vi "FT_Get_Device_Serial_Number_By_Index2011.vi"(0 "Device Index":u32) -> (1 "FT_Status":u32(ring) items=["FT_OK", "FT_INVALID_HANDLE", "FT_DEVICE_NOT_FOUND", "FT_DEVICE_NOT_OPENED", "FT_IO_ERROR", "FT_INSUFFICIENT_RESOURCES", "FT_INVALID_PARAMETER", "FT_INVALID_BAUD_RATE", "FT_DEVICE_NOT_OPENED_FOR_ERASE", "FT_DEVICE_NOT_OPENED_FOR_WRITE", "FT_FAILED_TO_WRITE_DEVICE", "FT_EEPROM_READ_FAILED", "FT_EEPROM_WRITE_FAILED", "FT_EEPROM_ERASE_FAILED", "FT_EEPROM_NOT_PRESENT", "FT_EEPROM_NOT_PROGRAMMED", "FT_INVALID_ARGS", "FT_NOT_SUPPORTED", "FT_OTHER_ERROR"], 2 "Device Serial Number":string)   [LabVIEW 2013]
uses:
  FTD2XX.dll
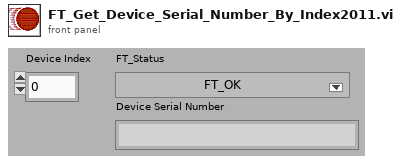
[diagram p1: front panel]
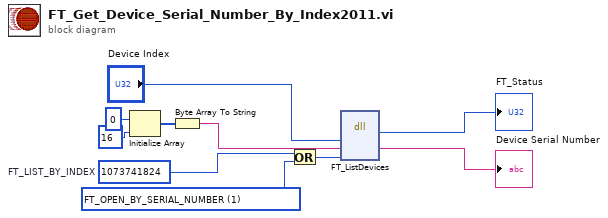
[diagram p0: block diagram]
diagram:
  w7 = u32 1 items=["FT_OPEN_BY_SERIAL_NUMBER"=1, "FT_OPEN_BY_DESCRIPTION"=2, "FT_OPEN_BY_LOCATION"=4] ("Flags")
  w6 = u32 1073741824  # FT_LIST_BY_INDEX
  n1 = Initialize Array(u8 0, 16 ("dimension size")) -> (w3:u8[])
  n2 = Byte Array To String(unsigned byte array=w3) -> (string=w2:string)
  n3 = Or(x=w6, y=w7) -> (x .or. y?=w5:u32)
  n4 = dll-call lib="FTD2XX.dll" fn="FT_ListDevices"("DeviceIndex"="Device Index", "DeviceDescription"=w2, "Flags"=w5) -> ("FT_Status"=→"FT_Status":u32, "DeviceDescription"=→"Device Serial Number":string)  [unwired: 5 in, 2 out]
